vi "TX_main.vi"() -> ()   [LabVIEW 2023]
uses:
  <vilib>/userDefined/High Color/IMAQdx.ctl
  TX_Control 3.ctl
  <vilib>/vision/Image Controls.llb/IMAQ Image.ctl
panel:
  in  "error in (no error) 2":errorcluster
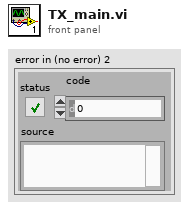
[diagram p1: front panel]
types:
  T1 = typedef "IMAQ Image.ctl" = refnum<image>
  T2 = typedef "TX_Control 3.ctl" = enum16{"Default", "StartCamera", "TakePhoto", "EnableTCP", "Cam2Display", "CloseAll"}
  T3 = cluster{"Enum":T2, "Data":variant, "Data2":variant}
  T4 = typedef "IMAQdx.ctl" = refnum<k21>
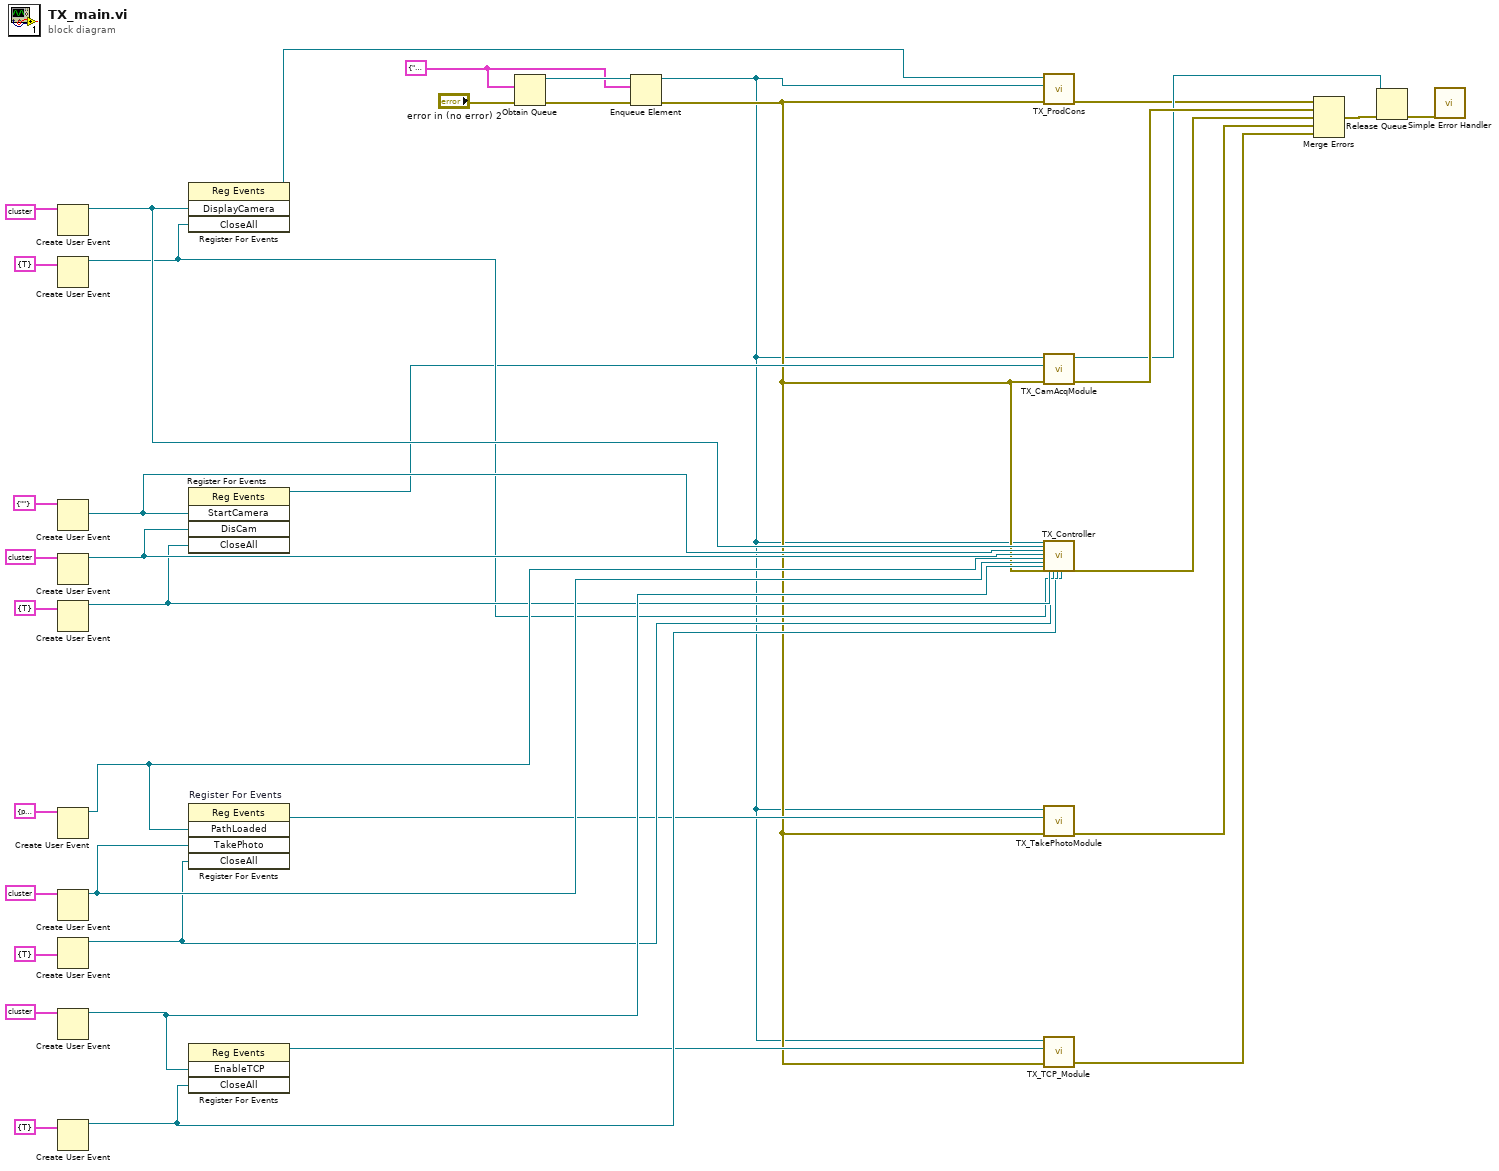
[diagram p0: block diagram]
diagram:
  w35 = T3 {"Enum"=enum."Default", "Data"=variant, "Data2"=variant(refnum<image> refnum)}
  n1 = Create User Event(user event datatype=cluster{"CamView":T1} {"CamView"=refnum} ("DisplayCamera")) -> (user event=w22:refnum<user-event>)  [unwired: 1 in, 1 out]
  n2 = Create User Event(user event datatype=cluster{"Boolean":bool} {"Boolean"=TRUE} ("CloseAll")) -> (user event=w15:refnum<user-event>)  [unwired: 1 in, 1 out]
  n3 = Create User Event(user event datatype=cluster{"CamSel":T4} {"CamSel"=""} ("StartCamera")) -> (user event=w21:refnum<user-event>)  [unwired: 1 in, 1 out]
  n4 = Create User Event(user event datatype=cluster{"CamView":T1} {"CamView"=refnum} ("DisCam")) -> (user event=w20:refnum<user-event>)  [unwired: 1 in, 1 out]
  n5 = Create User Event(user event datatype=cluster{"Boolean":bool} {"Boolean"=TRUE} ("CloseAll")) -> (user event=w16:refnum<user-event>)  [unwired: 1 in, 1 out]
  n6 = Create User Event(user event datatype=cluster{"File Path":path} {"File Path"=path ""} ("PathLoaded")) -> (user event=w19:refnum<user-event>)  [unwired: 1 in, 1 out]
  n7 = Create User Event(user event datatype=cluster{"CamView":T1} {"CamView"=refnum} ("TakePhoto")) -> (user event=w18:refnum<user-event>)  [unwired: 1 in, 1 out]
  n8 = Create User Event(user event datatype=cluster{"CloseAll":bool} {"CloseAll"=TRUE} ("CloseAll")) -> (user event=w14:refnum<user-event>)  [unwired: 1 in, 1 out]
  n9 = Create User Event(user event datatype=cluster{"CamView":T1} {"CamView"=refnum} ("EnableTCP")) -> (user event=w17:refnum<user-event>)  [unwired: 1 in, 1 out]
  n10 = Create User Event(user event datatype=cluster{"Boolean":bool} {"Boolean"=TRUE} ("CloseAll")) -> (user event=w13:refnum<user-event>)  [unwired: 1 in, 1 out]
  n11 = register-events(w22, w15) -> (reference out=w2:refnum<event-registration>)  [unwired: 2 in, 1 out]
  n12 = register-events(w21, w20, w16) -> (reference out=w6:refnum<event-registration>)  [unwired: 2 in, 1 out]
  n13 = register-events "Register For Events"(w19, w18, w14) -> (reference out=w11:refnum<event-registration>)  [unwired: 2 in, 1 out]
  n14 = register-events(w17, w13) -> (reference out=w9:refnum<event-registration>)  [unwired: 2 in, 1 out]
  n15 = Obtain Queue(element data type=w35, error in (no error)="error in (no error) 2") -> (queue out=w37:refnum<queue>, error out=w38:errorcluster)  [unwired: 3 in, 1 out]
  n16 = Enqueue Element(queue=w37, element=w35, error in (no error)=w38) -> (queue out=w3:refnum<queue>, error out=w4:errorcluster)  [unwired: 1 in, 1 out]
  n17 = call "TX_ProdCons.vi"("error in"=w4, "queue in"=w3, "Event Registration Refnum"=w2) -> ("error out"=w1:errorcluster)  [unwired: 8 in]
  n18 = call "TX_CamAcqModule.vi"("error out"=w4, "Event Registration Refnum"=w6, "queue out"=w3) -> ("error out 2"=w8:errorcluster, "queue out 2"=w7:refnum<queue>)  [unwired: 7 in]
  n19 = call "TX_Controller.vi"("queue out"=w3, "DisplayCamera"=w22, "StartCamera"=w21, "DisCam"=w20, "PathLoaded"=w19, "TakePhoto"=w18, "EnableTCP"=w17, "error out"=w4, "CloseAll"=w16, "CloseAll 2"=w15, "CloseAll 3"=w14, "CloseAll 4"=w13) -> ("error out 2"=w12:errorcluster)  [unwired: 15 in]
  n20 = call "TX_TakePhotoModule.vi"("error out"=w4, "Event Registration Refnum"=w11, "queue out"=w3) -> ("error out 2"=w10:errorcluster)  [unwired: 8 in]
  n21 = call "TX_TCP_Module.vi"("error out"=w4, "Event Registration Refnum"=w9, "queue out"=w3) -> ("error out 2"=w5:errorcluster)  [unwired: 8 in]
  n22 = Merge Errors(w1, w8, w12, w10, w5) -> (w33:errorcluster)
  n23 = Release Queue(queue=w7, error in (no error)=w33) -> (error out=w34:errorcluster)  [unwired: 1 in, 2 out]
  n24 = call <vilib>:"Simple Error Handler.vi"("error in (no error)"=w34) -> ()  [unwired: 4 in, 5 out]
